vi "Run All.vi"(8 "Error In":errorcluster) -> (0 "Error Out":errorcluster)   [LabVIEW 2018, in "Tests.lvlib" / "Compile.lvlib"]
uses:
  Compile.lvlib
  <vilib>/addons/_JKI Toolkits/Caraya/classes/Test/Test.lvclass
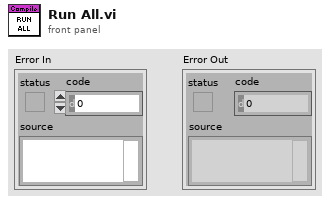
[diagram p1: front panel]
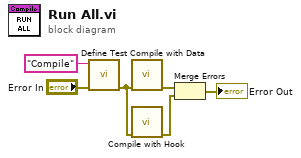
[diagram p0: block diagram]
diagram:
  n1 = call <vilib>:"Define Test.vi"("error in (no error)"="Error In", "Label (VI Title)"="Compile") -> ("error out"=w1:errorcluster)  [unwired: 9 in]
  n2 = call "Compile with Data.vi"("Error In"=w1) -> ("Error Out"=w4:errorcluster)  [unwired: 10 in]
  n3 = call "Compile with Hook.vi"("Error In"=w1) -> ("Error Out"=w2:errorcluster)  [unwired: 10 in]
  n4 = Merge Errors(w4, w2) -> (→"Error Out":errorcluster)
